vi "Log Queue.vi"() -> (1 "Log Queue":refnum<queue>)   [LabVIEW 2015]
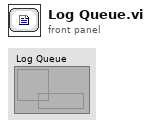
[diagram p1: front panel]
types:
  T1 = cluster{"Log Level":enum16{"INFO", "DEBUG", "WARN", "ERROR"}, "Time Stamp":timestamp, "Call Chain":string[], "Message":string}
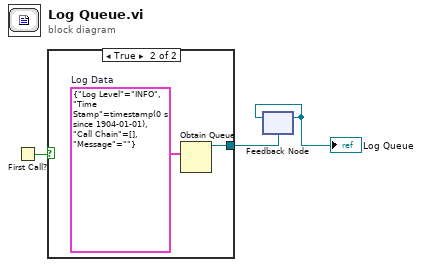
[diagram p0: block diagram]
diagram:
  n1 = First Call?() -> (First Call?: T/F=w2:bool)
  n2 = case shown="True" w2 {
    tunnel: [_ w5] -> w3
    frame False {
    }
    frame True {
      w4 = T1 {"Log Level"=enum."INFO", "Time Stamp"=timestamp(0 s since 1904-01-01), "Call Chain"=[], "Message"=""}  # Log Data
      n3 = Obtain Queue(element data type=w4) -> (queue out=w5:refnum<queue>)  [unwired: 4 in, 2 out]
    }
  }
  n4 = feedback #1(w3) -> (w1:refnum<queue>)
  "Log Queue" <- w1
  n5 = feedback-in #1(w1) -> ()
